vi "LEBITplc.CreateEvents.vi"(0 "i ref in":refnum<vi>, 2 "i attribute in":T1, 5 "error in":errorcluster) -> (14 "i ref out":refnum<vi>, 16 "i attribute out":T1, 19 "error out":errorcluster)   [LabVIEW 2014, in "LEBITplc.lvlib"]
uses:
  LEBITplc.lvlib
  LEBITplc.i attribute.ctl
  CS_Core/BaseProcess/BaseProcess.event definition.ctl
  CS_Core/CAEObj/CAEObj.event definition.ctl
  CS_Core/BaseProcess/BaseProcess.descriptor string definition.ctl
  CS_Core/BaseProcess/BaseProcess.lvlib
  CS_Core/CAEObj/CAEObj.lvlib
panel:
  in  "CAEEvtDef":T2
  in  "event definition":T3
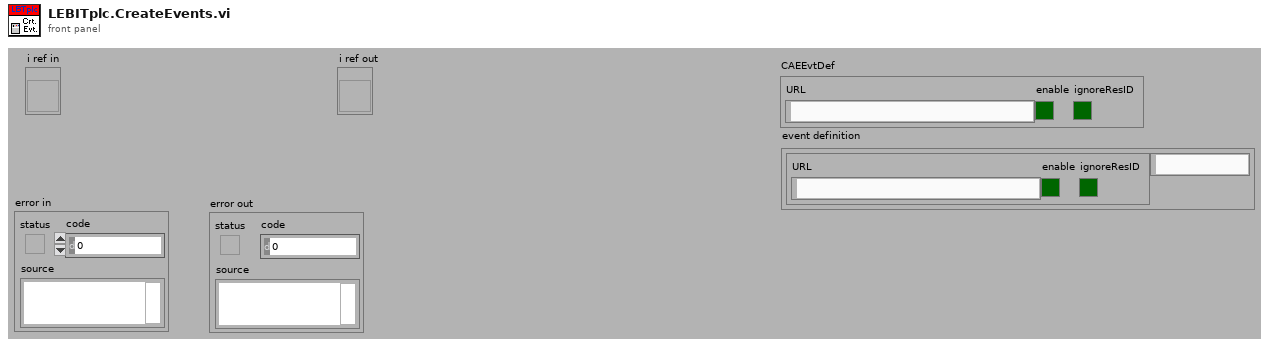
[diagram p1: front panel]
types:
  T1 = typedef "LEBITplc.lvlib/LEBITplc.i attribute.ctl" = cluster{"LLFLocation":string, "SetFileLocation":string, "nickNames":string[], "setValuePLCServiceID":i32[], "GUIServiceID":i32[], "monValuePLC":string[], "SetValueServiceID":i32[], "MonValueServiceID":i32[], "SetValue":dbl[][], "SetValueMin":dbl[], "SetValueMax":dbl[], "SetValueInfoServiceID":i32[], "GUINames":string[], "ListOfBases":string[], "Scale":dbl[], "Offset":dbl[], "setValuePLC":string[], "BaseName":string[], "ScaleServiceID":i32[], "OffsetServiceID":i32[], "AllPLCValues":string[], "CondSpecialArray":string[][], "CondSpecialIndex":i32[], "CondSpecialMonValue":dbl[], "RecentlyChanged":i32[], "SetFileLocationID":i32, "Dependent-Monitors":string[][], "LastLoadedFiles":string[], "IonGuideCalibLocation":string, "Monitor Dependent":string[], "Special":string[], "PLC?":bool[], "Start Date":string, "ListOfBasesServiceID":i32, "SETRA VISA resource":refnum<visa-resource-name>}
  T2 = typedef "CAEObj.lvlib/CAEObj.event definition.ctl" = cluster{"URL":string, "enable":bool, "ignoreResID":bool}
  T3 = typedef "BaseProcess.lvlib/BaseProcess.event definition.ctl" = cluster{"CAEEvtDef":T2, "Data Descriptor":T4}
  T4 = typedef "BaseProcess.lvlib/BaseProcess.descriptor string definition.ctl" = string
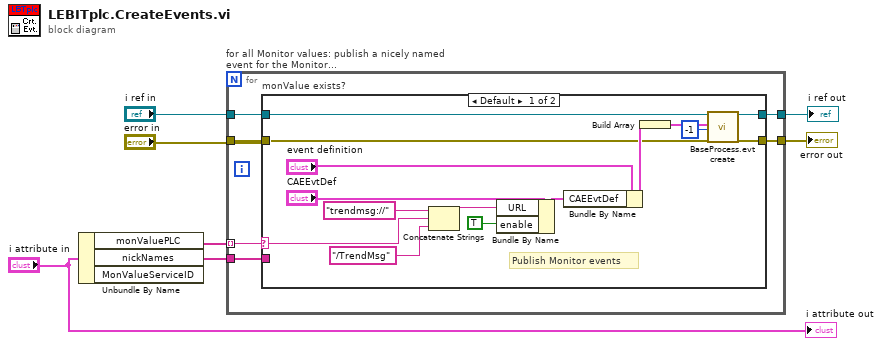
[diagram p0: block diagram]
diagram:
  n1 = Unbundle By Name("i attribute in") -> ("monValuePLC"=w1:string[], "nickNames"=w4:string[])  [unwired: 1 out]
  n2 = for "for all Monitor values: publish a nicely named event for the Monitor..." {
    tunnel: w1 -> [w13] mode=indexing
    tunnel: w4 -> [w12]
    tunnel: "i ref in" -> [w11]
    tunnel: "error in" -> [w10]
    tunnel: [w9] -> w6
    tunnel: [w8] -> w5
    n3 = case "monValue exists?" shown="Default" w13 {
      selector: w13 -> [w19 _]
      tunnel: w12 -> [_ _]
      tunnel: w11 -> [w24 w30]
      tunnel: w10 -> [w23 w29]
      tunnel: [w21 w29] -> w9
      tunnel: [w22 w30] -> w8
      frame Default {
        # "Publish Monitor events"
        n4 = Concatenate Strings("trendmsg://" ("string"), w19, "/TrendMsg" ("string")) -> (w17:string)
        n5 = Bundle By Name(cluster="CAEEvtDef", "URL"=w17, "enable"=TRUE) -> (w26:T2)
        n6 = Bundle By Name(cluster="event definition", "CAEEvtDef"=w26) -> (w27:T3)
        n7 = Build Array(w27) -> (w28:T3[])
        n8 = call "BaseProcess.evt create.vi"("i ref in"=w24, "newEvents"=w28, "ms timeout (10000)"=-1, "error in (no error)"=w23) -> ("i ref out"=w22:refnum<vi>, "error out"=w21:errorcluster)  [unwired: 12 in, 2 out]
      }
      frame "" {
      }
    }
  }
  "error out" <- w6
  "i ref out" <- w5
  "i attribute out" <- "i attribute in"
